vi "DelayGeneratorGetOffset.vi"(9 "error in (no error)":errorcluster) -> (2 "Offset":dbl[unit] format="%.6g", 6 "error out":errorcluster)   [LabVIEW 2009]
uses:
  Controls/DelayTarget.ctl
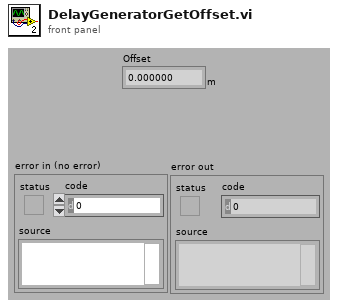
[diagram p1: front panel]
types:
  T1 = typedef "DelayTarget.ctl" = cluster{"Time":timestamp, "Position":dbl[unit], "Velocity":dbl[unit]}
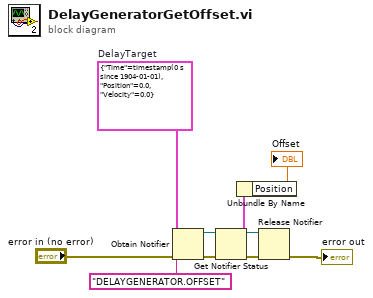
[diagram p0: block diagram]
diagram:
  w3 = T1 {"Time"=timestamp(0 s since 1904-01-01), "Position"=0.0, "Velocity"=0.0}  # DelayTarget
  n1 = Obtain Notifier(name (unnamed)="DELAYGENERATOR.OFFSET", notification data type=w3, error in (no error)="error in (no error)") -> (notifier out=w8:refnum<notifier>, error out=w4:errorcluster)  [unwired: 1 in, 1 out]
  n2 = Get Notifier Status(notifier=w8, error in (no error)=w4) -> (notifier out=w5:refnum<notifier>, current notification=w2:T1, error out=w6:errorcluster)  [unwired: 2 out]
  n3 = Unbundle By Name(w2) -> ("Position"=→"Offset":dbl[unit])
  n4 = Release Notifier(notifier=w5, error in (no error)=w6) -> (error out=→"error out":errorcluster)  [unwired: 1 in, 2 out]
